vi "Control_GEA2_Loop.vi"(0 "GEA2":refnum<queue>, 2 "Command (ERD Loop Control)":T1, 11 "Error In":errorcluster) -> (15 "Error Out":errorcluster)   [LabVIEW 2014]
uses:
  Utility/Labview GEA2 Toolkit v2.1/GExplorer Support/typedefs/GExplorer_Data_Cluster.ctl
  type defs/GEA2_Control_Command.ctl
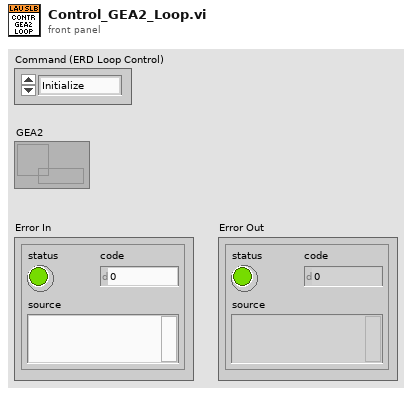
[diagram p1: front panel]
types:
  T1 = typedef "GEA2_Control_Command.ctl" = enum16{"Initialize", "Shutdown"}
  T2 = typedef "GExplorer_Data_Cluster.ctl" = cluster{"Data":variant, "State":enum16{"Add to Log", "Clear", "Shutdown"}}
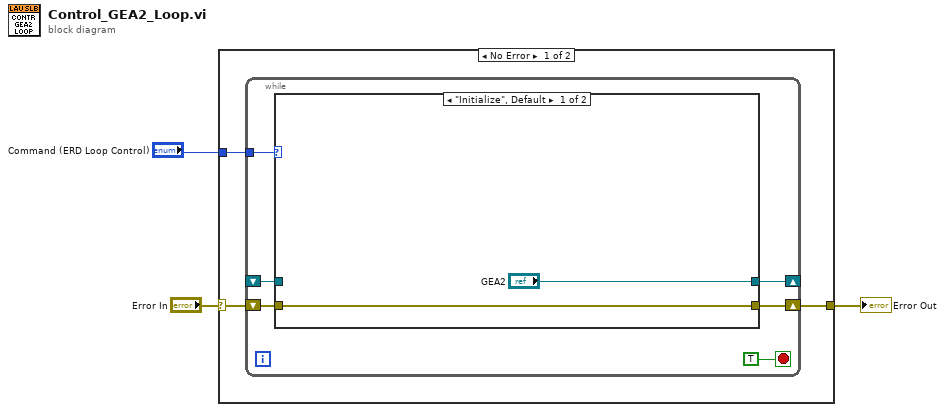
[diagram p0: block diagram]
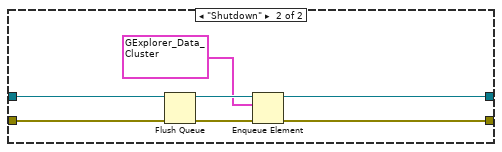
[diagram p2: hidden frame]
diagram:
  n1 = case shown="No Error" "Error In" {
    selector: "Error In" -> [w5 w22]
    tunnel: "Command (ERD Loop Control)" -> [w6 _]
    tunnel: [w4 w22] -> w2
    frame No Error {
      n2 = while {
        tunnel: w6 -> [w12]
        shift-right: [w9] -> w4
        shift-left: w5 -> [w10]
        shift-right: [w8] -> _
        shift-left: _ -> [w7]
        stop <- TRUE stop-if-true
        n3 = case shown="\"Initialize\", Default" w12 {
          tunnel: w10 -> [w14 w21]
          tunnel: [w14 w18] -> w9
          tunnel: ["GEA2" w17] -> w8
          tunnel: w7 -> [_ w20]
          frame "Initialize", Default {
          }
          frame "Shutdown" {
            n4 = Flush Queue(queue=w20, error in (no error)=w21) -> (queue out=w16:refnum<queue>, error out=w19:errorcluster)  [unwired: 1 out]
            n5 = Enqueue Element(queue=w16, element=T2 {"Data"=variant, "State"=enum."Shutdown"}, error in (no error)=w19) -> (queue out=w17:refnum<queue>, error out=w18:errorcluster)  [unwired: 1 in, 1 out]
          }
        }
      }
    }
    frame Error {
    }
  }
  "Error Out" <- w2
